vi "Management_Init.vi"(7 "error in (no error)":errorcluster, 9 "LAW":T1, 10 "object in":refnum<class "Display.lvclass">) -> (0 "error out":errorcluster, 3 "object out":refnum<class "Display.lvclass">)   [LabVIEW 2015, in "UserManagement.lvlib" / "Display.lvclass"]
uses:
  Display.lvclass
  _typedef/userOfLoginLaw.ctl
  Display.lvclass/Display.ctl
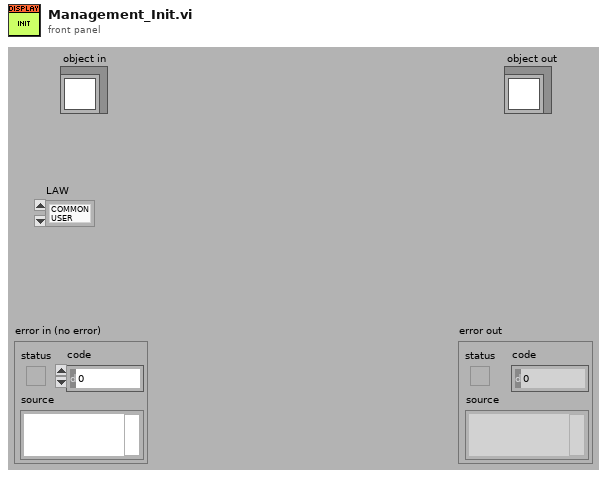
[diagram p1: front panel]
types:
  T1 = typedef "userOfLoginLaw.ctl" = enum16{"COMMONUSER", "ADMIN"}
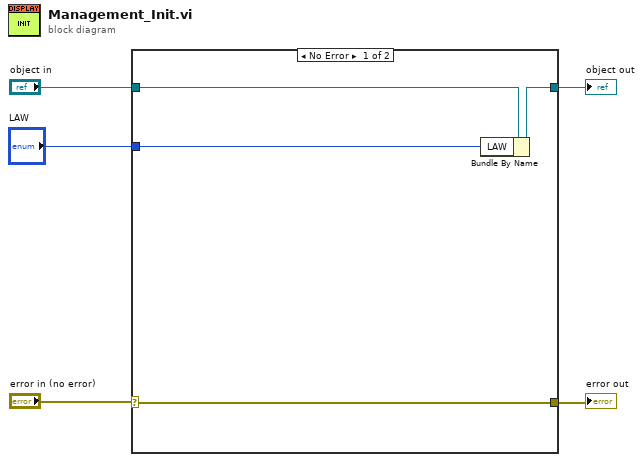
[diagram p0: block diagram]
diagram:
  n1 = case shown="No Error" "error in (no error)" {
    selector: "error in (no error)" -> [w7 w10]
    tunnel: "object in" -> [w9 w11]
    tunnel: [w8 w11] -> w4
    tunnel: [w7 w10] -> w2
    tunnel: "LAW" -> [w6 _]
    frame No Error {
      n2 = Bundle By Name(cluster=w9, "LAW"=w6) -> (w8:refnum<class "Display.lvclass">)
    }
    frame Error {
    }
  }
  "object out" <- w4
  "error out" <- w2
